vi "Dequeue and Destroy.vi"(8 "error in (no error)":errorcluster, 10 "Timeout (ms)":i32, 11 "Reply Queue In":refnum<queue>) -> (0 "error out":errorcluster, 2 "Timed Out?":bool, 3 "Event Cluster Out":T1)   [LabVIEW 2017, in "Broadcast Actor.lvlib" / "Broadcast Actor.lvclass"]
uses:
  Broadcast Actor.lvclass
  Type Defs/Events Type Def.ctl
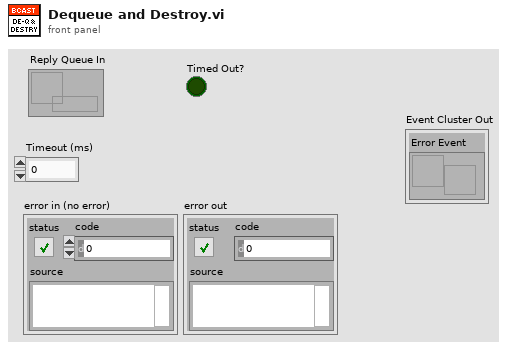
[diagram p1: front panel]
types:
  T1 = typedef "Broadcast Actor.lvlib/Broadcast Actor.lvclass/Events Type Def.ctl" = cluster{"Error Event":refnum<user-event>}
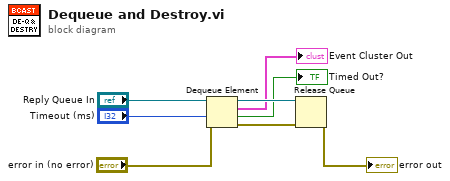
[diagram p0: block diagram]
diagram:
  n1 = Dequeue Element(queue="Reply Queue In", timeout in ms (-1)="Timeout (ms)", error in (no error)="error in (no error)") -> (queue out=w4:refnum<queue>, element=→"Event Cluster Out":T1, timed out?=→"Timed Out?":bool, error out=w5:errorcluster)
  n2 = Release Queue(queue=w4, error in (no error)=w5) -> (error out=→"error out":errorcluster)  [unwired: 1 in, 2 out]
